vi "Teleop.vi"(10 "Match Info":T1={"Autonomous Elapsed Seconds"=0.0, "TeleOp Elapsed Seconds"=0.0, "Disabled Elapsed Seconds"=0.0, "Visited Autonomous"=FALSE, "Visited TeleOp"=FALSE, "Visited Disabled"=FALSE, "Autonomous Settings"={"Autonomous Style"=enum."Independent", "VI Refnum"=refnum}}, 11 "Call Context":T2) -> ()   [LabVIEW 2016]
doc: "This VI is called for each TeleOp packet received from the DS where the robot is not disabled. It is often used to read from the joysticks and update I/O or to update setpoints for timed control loops. It should complete and return within 20 milliseconds or it may miss DS packets."
uses:
  <vilib>/Rock Robotics/WPI/DriverStation/WPI_DriverStationDerivedRobotMode.ctl
  <vilib>/Rock Robotics/WPI/DriverStation/WPI_DriverStationMatch Info.ctl
  <vilib>/Rock Robotics/WPI/ThirdParty/CanMotor/TalonSRX/WPI_CANTalonSRX_APIControlMode.ctl
  <vilib>/Rock Robotics/WPI/Utilities/WPI_GetSetVariantRefNum.vi
  <vilib>/Rock Robotics/Network Tables/NT Write Boolean.vi
  <vilib>/Rock Robotics/Network Tables/NT Write Boolean Array.vi
  <vilib>/Rock Robotics/Network Tables/NT Write Numeric Array.vi
  <vilib>/Rock Robotics/WPI/Solenoid/Deprecated/WPI_SolenoidSetBool.vi
  <vilib>/Rock Robotics/WPI/Ultrasonic/WPI_SonarMB1010AnalogRefNum Registry Get.vi
  <vilib>/Rock Robotics/WPI/Ultrasonic/WPI_SonarMB1010AnalogGetRange.vi
  <vilib>/Rock Robotics/Network Tables/NT Read Number.vi
  <vilib>/Rock Robotics/Network Tables/NT Write Number.vi
panel:
  out "element":dbl
  out "upper limit":dbl
  out "gyro":dbl
  out "sonar distance (inches)":dbl
  out "Encoder Loop 2":string
  out "Encoder Loop":dbl
  out "Encoder Rate":dbl
  out "Encoder State":string
  out "Encoder Direction":string
  out "Distance 2":dbl
  out "Angle 2":dbl
  out "Distance":dbl
  out "Enabled":bool
  out "Compressor Running":bool
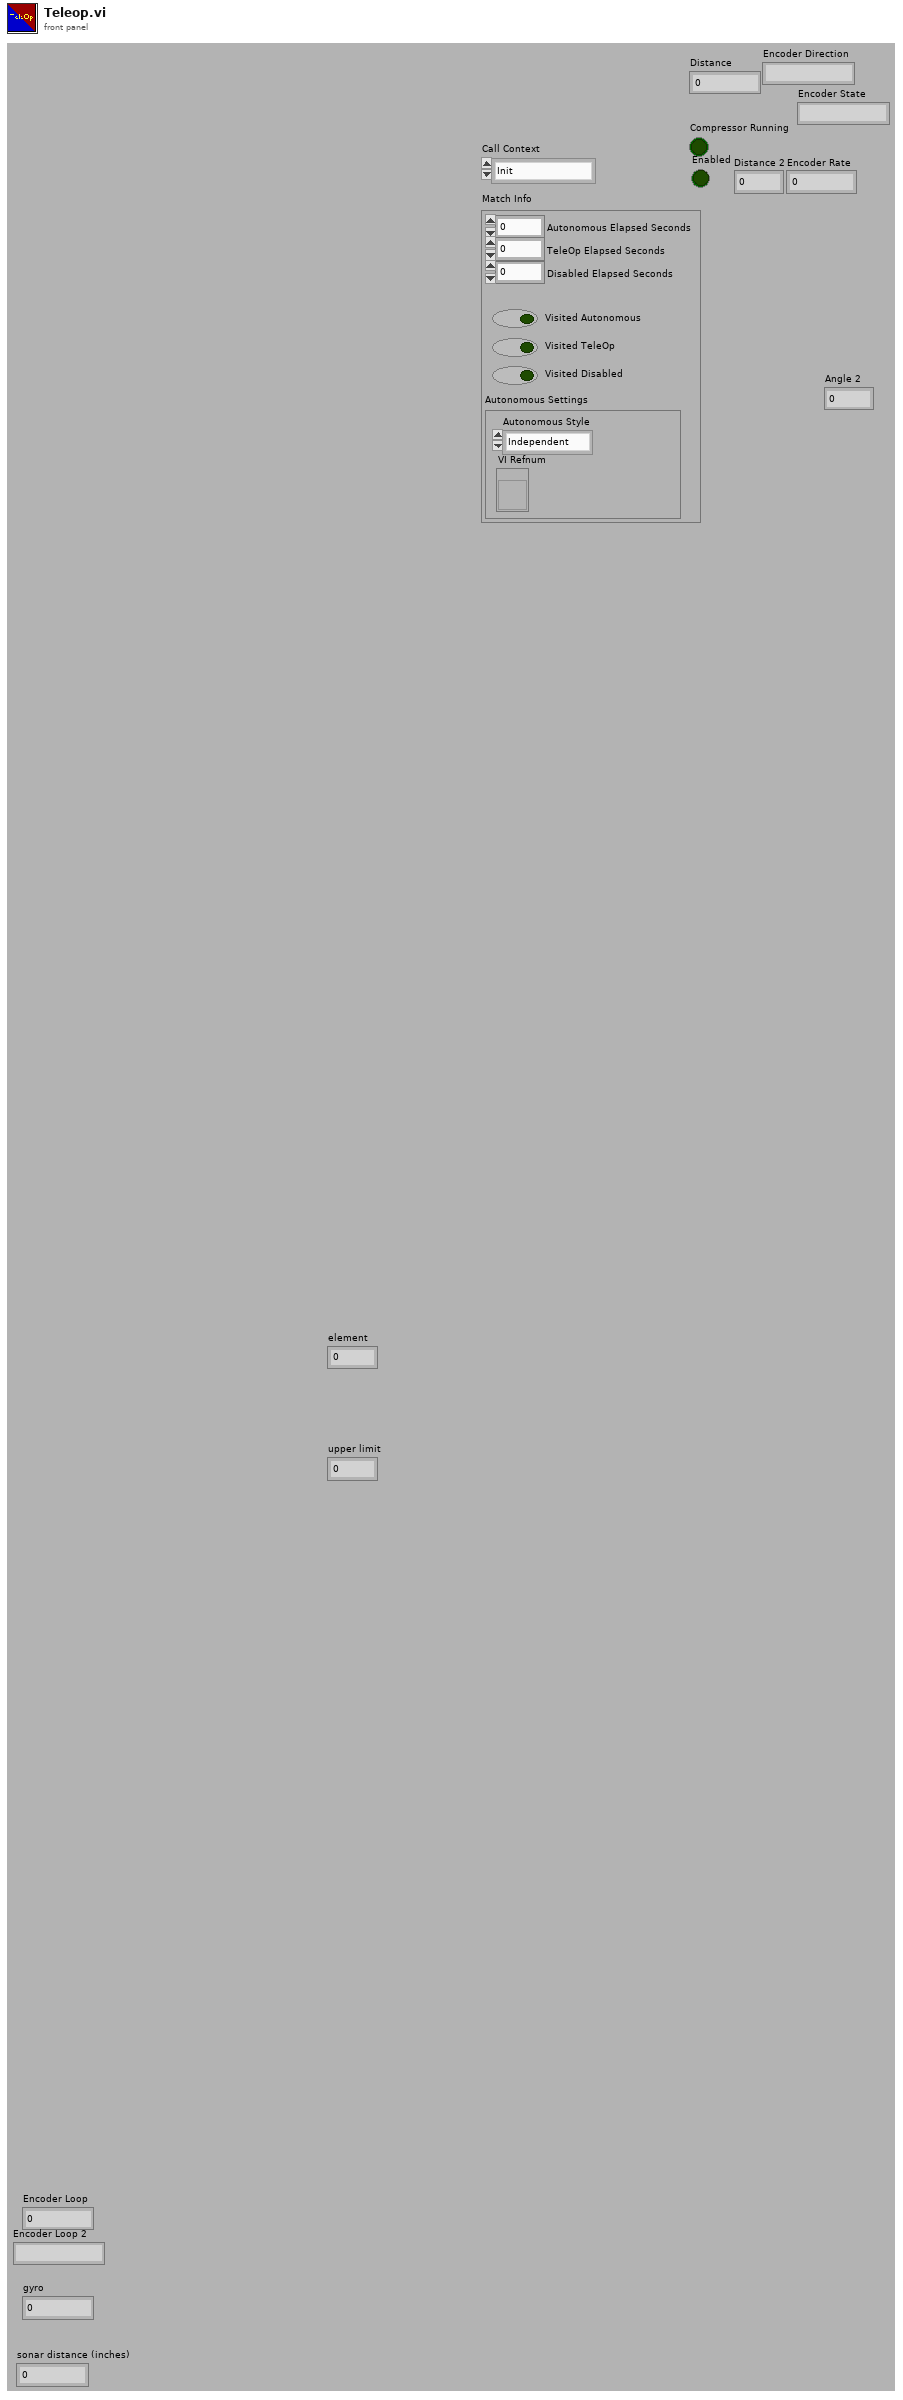
[diagram p1: front panel]
types:
  T1 = typedef "WPI_DriverStationMatch Info.ctl" = cluster{"Autonomous Elapsed Seconds":dbl, "TeleOp Elapsed Seconds":dbl, "Disabled Elapsed Seconds":dbl, "Visited Autonomous":bool, "Visited TeleOp":bool, "Visited Disabled":bool, "Autonomous Settings":cluster{"Autonomous Style":enum16{"Iterative", "Independent"}, "VI Refnum":refnum<vi>}}
  T2 = typedef "WPI_DriverStationDerivedRobotMode.ctl" = enum16{"Init", "Execute", "Stop"}
  T3 = typedef "WPI_EncoderDevRef.ctl" = cluster{"DevStatus":errorcluster, "EncoderIndex":T4, "CounterIndex":T5, "DistancePerCount":dbl, "Decoding Type":T6}
  T4 = typedef "FPGA_EncoderIdx.ctl" = enum8{"Enc 0", "Enc 1", "Enc 2", "Enc 3", "Enc 4", "Enc 5", "Enc 6", "Enc 7", "Invalid"}
  T5 = typedef "FPGA_CounterCtrSystemIndex.ctl" = enum8{"Ctr 0", "Ctr 1", "Ctr 2", "Ctr 3", "Ctr 4", "Ctr 5", "Ctr 6", "Ctr 7", "Invalid"}
  T6 = typedef "WPI_EncoderType.ctl" = enum16{"1x", "2x", "4x"}
  T7 = typedef "WPI_JoystickDevRef.ctl" = cluster{"Device":T8}
  T8 = typedef "WPI_JoystickDeviceEnum.ctl" = enum16{"USB 0", "USB 1", "USB 2", "USB 3", "USB 4", "USB 5"}
  T9 = typedef "WPI_GyroDevRef.ctl" = cluster{"DevStatus":errorcluster, "Analog Channel":T10, "Offset":dbl, "Gain (VoltsPerDegree/Second)":dbl, "Gyro Type":enum16{"Analog", "XRS450"}, "Handle":i32, "SPI Bus":T11, "Device Found":bool, "Sample Rate":dbl, "Calibrate On Open":bool}
  T10 = typedef "FPGA_AIChannel.ctl" = enum8{"AI 0", "AI 1", "AI 2", "AI 3", "AI MXP 0", "AI MXP 1", "AI MXP 2", "AI MXP 3", "Invalid"}
  T11 = typedef "spi_bus.ctl" = enum16{"SPI On-Board, CS0", "SPI On-Board, CS1", "SPI On-Board, CS2", "SPI On-Board, CS3", "SPI MXP", "Invalid"}
  T12 = typedef "WPI_SonarMB1010AnalogDeviceRef.ctl" = cluster{"AIDeviceRef":T13, "Scaling factor (V/in)":dbl, "Average Bits":u8}
  T13 = typedef "WPI_AnalogChannelDevRef.ctl" = cluster{"DevStatus":errorcluster, "Analog Channel":T10}
  T14 = typedef "WPI_CompressorDevRef.ctl" = cluster{"DevStatus":errorcluster, "Pneumatics Control Module":u8}
  T15 = typedef "WPI_SolenoidDevRef.ctl" = cluster{"DevStatus":errorcluster, "Pneumatics Control Module":u8, "Forward Solenoid Channel":T16, "Reverse Solenoid Channel":T16}
  T16 = typedef "WPI_SolenoidChannel.ctl" = enum8{"Solenoid 0", "Solenoid 1", "Solenoid 2", "Solenoid 3", "Solenoid 4", "Solenoid 5", "Solenoid 6", "Solenoid 7", "Invalid"}
  T17 = typedef "WPI_MotorControlDeviceRef.ctl" = cluster{"DeviceStatus":errorcluster, "Type":T18, "PWM":cluster{"PWM Channel":T19, "DeadBand":T20}, "CAN":cluster{"Device Number":u8, "SetOutput VI Ref":variant, "GetOutput VI Ref":variant, "Enable VI Ref":variant, "Disable VI Ref":variant, "Data":variant}, "Invert":bool}
  T18 = typedef "WPI_MotorControlType.ctl" = enum16{"PWM", "CAN"}
  T19 = typedef "FPGA_DIOPWMChannel.ctl" = enum8{"PWM 0", "PWM 1", "PWM 2", "PWM 3", "PWM 4", "PWM 5", "PWM 6", "PWM 7", "PWM 8", "PWM 9", "PWM MXP 0", "PWM MXP 1", "PWM MXP 2", "PWM MXP 3", "PWM MXP 4", "PWM MXP 5", "PWM MXP 6", "PWM MXP 7", "PWM MXP 8", "PWM MXP 9", "Invalid"}
  T20 = typedef "WPI_PWMDeadband.ctl" = cluster{"Name":string, "maxPositivePwm":i32, "minPositivePwm":i32, "centerPwm":i32, "maxNegativePwm":i32, "minNegativePwm":i32, "angularRange":u16}
  T21 = typedef "WPI_CANTalonSRX_APIControlMode.ctl" = enum8{"Percent VBus", "Speed", "Position", "Slave", "Unchanged / Invalid", "Voltage Compensation", "Current", "Motion Profile", "Motion Magic"}
  T22 = typedef "WPI_RobotDriveDevRef.ctl" = cluster{"DevStatus":errorcluster, "Motors[]":T17[], "Square Inputs":bool, "Max Output":dbl}
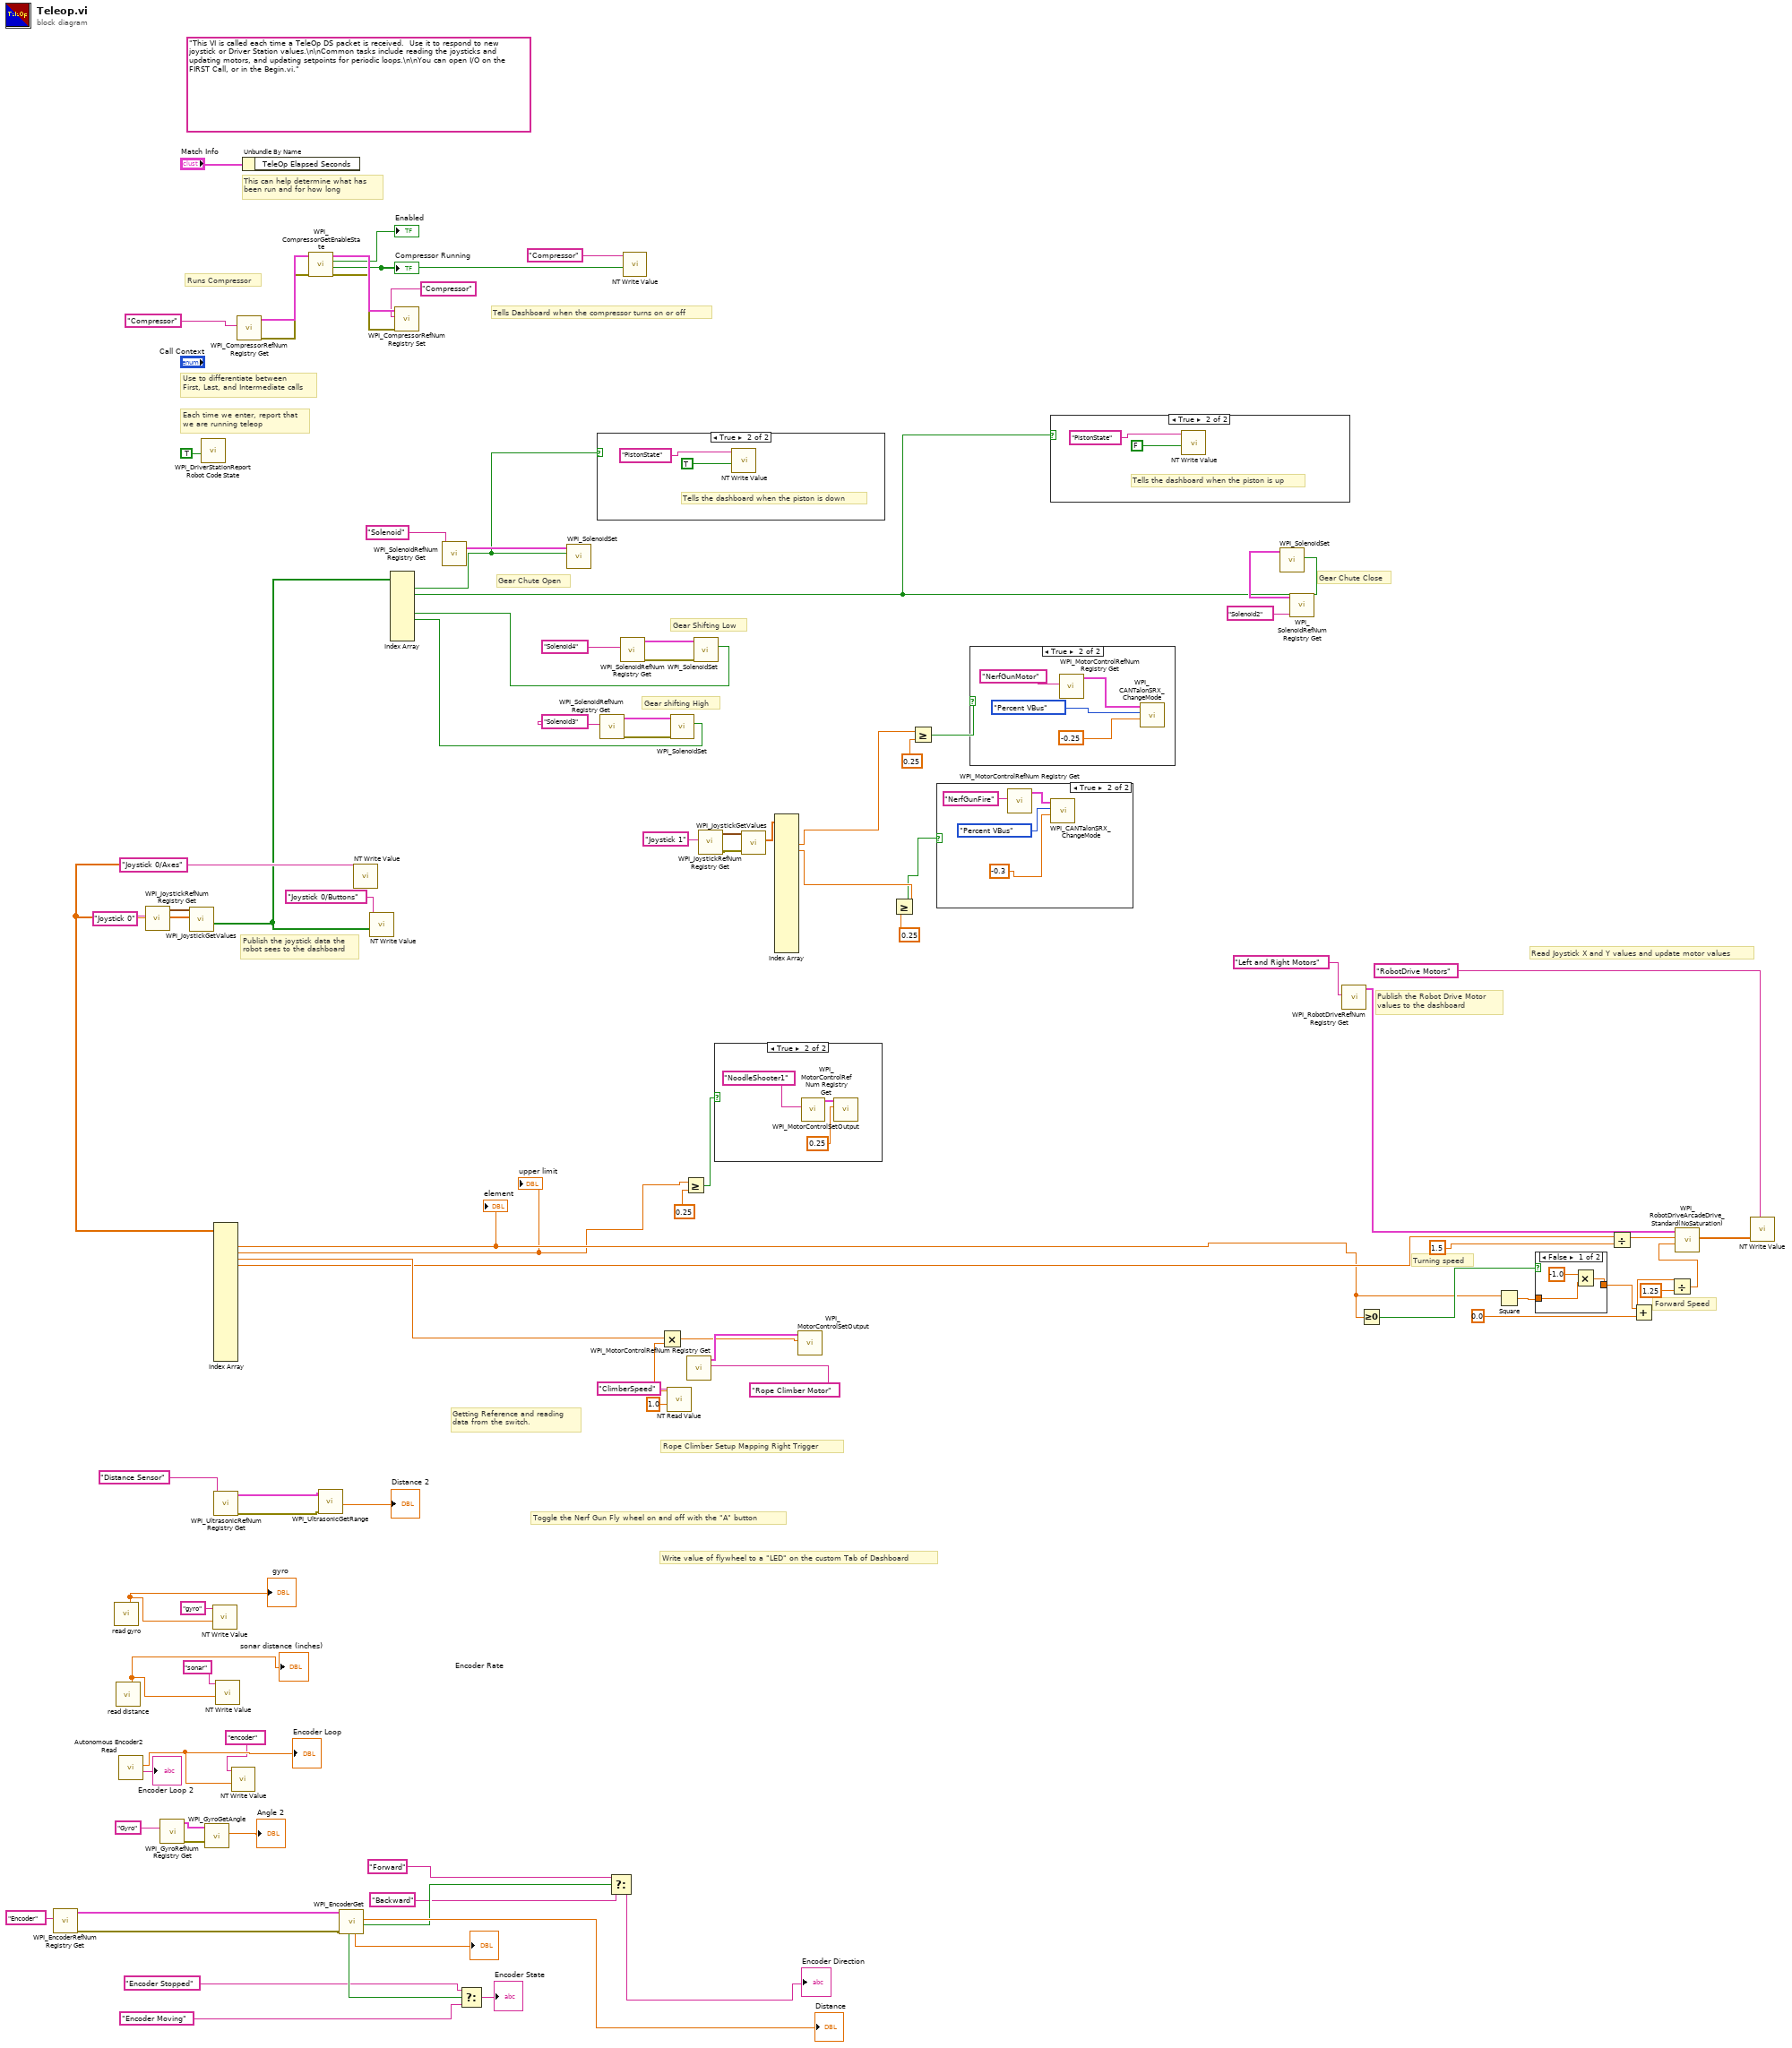
[diagram p0: block diagram]
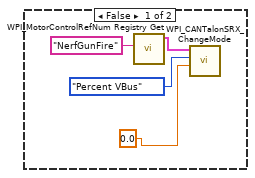
[diagram p2: hidden frame]
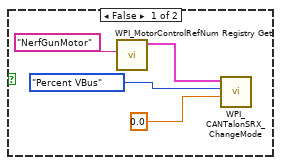
[diagram p3: hidden frame]
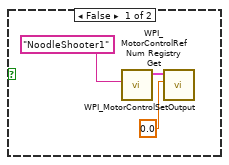
[diagram p4: hidden frame]
diagram:
  (unwired) "This VI is called each time a TeleOp DS packet is received.  Use it to respond to new joystick or Driver Station values.\n\nCommon tasks include reading the joysticks and updating motors, and updating setpoints for periodic loops.\n\nYou can open I/O on the FIRST Call, or in the Begin.vi."
  # "Write value of flywheel to a \"LED\" on the custom Tab of Dashboard"
  # "Toggle the Nerf Gun Fly wheel on and off with the \"A\" button"
  # "Gear Chute Open"
  # "Gear Chute Close"
  # "Gear shifting High"
  # "Gear Shifting Low"
  # "Turning speed"
  # "Forward Speed"
  # "Rope Climber Setup Mapping Right Trigger"
  # "Getting Reference and reading \ndata from the switch."
  # "Publish the joystick data the\nrobot sees to the dashboard"
  # "Publish the Robot Drive Motor\nvalues to the dashboard"
  # "Read Joystick X and Y values and update motor values"
  # "Tells Dashboard when the compressor turns on or off"
  # "Runs Compressor"
  # "Each time we enter, report that\nwe are running teleop"
  # "Use to differentiate between\nFirst, Last, and Intermediate calls"
  # "This can help determine what has\nbeen run and for how long"
  n1 = call <vilib>:"WPI_EncoderRefNum Registry Get.vi"("refnum name"="Encoder") -> ("error out"=w63:errorcluster, "EncoderDevRef"=w64:T3)  [unwired: 9 in]
  n2 = call "read gyro.vi"() -> ("Angle 2"=w36:dbl)  [unwired: 10 in, 1 out]
  "gyro" <- w36
  n3 = call "read distance.vi"() -> ("Distance 2"=w34:dbl)  [unwired: 10 in, 1 out]
  "sonar distance (inches)" <- w34
  n4 = call "Autonomous Encoder2 Read.vi"() -> ("Encoder Direction"=→"Encoder Loop 2":string, "Encoder Distance"=w31:dbl)  [unwired: 9 in, 1 out]
  "Encoder Loop" <- w31
  n5 = call <vilib>:"WPI_JoystickRefNum Registry Get.vi"("refnum name"="Joystick 0") -> ("JoystickDevRef"=w80:T7)  [unwired: 1 in, 9 out]
  n6 = call <vilib>:"WPI_GyroRefNum Registry Get.vi"("refnum name"="Gyro") -> ("error out"=w58:errorcluster, "GyroDevRef"=w59:T9)  [unwired: 9 in]
  n7 = call <vilib>:"WPI_JoystickGetValues.vi"("JoystickDevRef"=w80) -> ("Buttons"=w74:bool[], "Axes"=w77:dbl[])  [unwired: 6 in, 3 out]
  n8 = call <vilib>:"WPI_DriverStationReport Robot Code State.vi"("TeleOp"=TRUE ("Autonomous")) -> ()  [unwired: 10 in, 1 out]
  n9 = call <vilib>:"WPI_GyroGetAngle.vi"("error in"=w58, "GyroDevRef"=w59) -> ("Angle"=→"Angle 2":dbl)  [unwired: 5 in, 4 out]
  n10 = call-poly <vilib>:"NT Write Value.vi"("Numeric"=w36, "Name"="gyro") -> ()  [unwired: 9 in, 1 out]
  n11 = Index Array(array=w77) -> (element #2=w29:dbl, element #3=w9:dbl, element #4=w68:dbl, element #5=w44:dbl)  [unwired: 20 in, 16 out]
  "upper limit" <- w9
  "element" <- w29
  n12 = call-poly <vilib>:"WPI_UltrasonicRefNum Registry Get.vi"("refnum name"="Distance Sensor") -> ("error out"=w54:errorcluster, "SonarMB1010AnalogDevRef"=w56:T12)  [unwired: 9 in]
  n13 = call-poly <vilib>:"NT Write Value.vi"("Numeric"=w34, "Name"="sonar") -> ()  [unwired: 9 in, 1 out]
  n14 = call-poly <vilib>:"NT Write Value.vi"("Numeric"=w31, "Name"="encoder") -> ()  [unwired: 9 in, 1 out]
  n15 = call <vilib>:"WPI_CompressorRefNum Registry Get.vi"("refnum name"="Compressor") -> ("error out"=w90:errorcluster, "CompressorDevRef"=w92:T14)  [unwired: 9 in]
  n16 = Unbundle By Name("Match Info") -> ()  [unwired: 1 out]
  n17 = call <vilib>:"WPI_CompressorGetEnableState.vi"("error in (no error)"=w90, "CompressorDevRef"=w92) -> ("error out"=w89:errorcluster, "Compressor Running"=w84:bool, "Enabled"=→"Enabled":bool, "CompressorDevRef"=w91:T14)  [unwired: 6 in]
  "Compressor Running" <- w84
  n18 = call-poly <vilib>:"WPI_UltrasonicGetRange.vi"("error in"=w54, "SonarMB1010AnalogDevRef"=w56) -> ("Distance"=→"Distance 2":dbl)  [unwired: 7 in, 2 out]
  n19 = call <vilib>:"WPI_EncoderGet.vi"("error in (no error)"=w63, "EncoderDevRef"=w64) -> ("Direction"=w53:bool, "Distance"=→"Distance":dbl, "Rate"=→"Encoder Rate":dbl, "Stopped"=w49:bool)  [unwired: 4 in, 2 out]
  n20 = call-poly <vilib>:"NT Write Value.vi"("Numeric Array"=w77, "Name"="Joystick 0/Axes") -> ()  [unwired: 9 in, 1 out]
  n21 = call-poly <vilib>:"NT Write Value.vi"("Boolean Array"=w74, "Name"="Joystick 0/Buttons") -> ()  [unwired: 9 in, 1 out]
  n22 = Index Array(array=w74) -> (element #1=w69:bool, element #2=w10:bool, element #5=w21:bool, element #6=w22:bool)  [unwired: 9 in, 5 out]
  n23 = call <vilib>:"WPI_CompressorRefNum Registry Set.vi"("error in (no error)"=w89, "refnum name"="Compressor", "CompressorDevRef"=w91) -> ()  [unwired: 7 in, 2 out]
  n24 = call <vilib>:"WPI_SolenoidRefNum Registry Get.vi"("refnum name"="Solenoid") -> ("SolenoidDevRef"=w70:T15)  [unwired: 9 in, 1 out]
  n25 = Select(t="Encoder Stopped", s=w49, f="Encoder Moving") -> (s? t:f=→"Encoder State":string)
  n26 = call-poly <vilib>:"WPI_SolenoidSet.vi"("Value"=w69, "SolenoidDevRef"=w70) -> ()  [unwired: 8 in, 2 out]
  n27 = case shown="True" w69 {
    frame False {
    }
    frame True {
      # "Tells the dashboard when the piston is down"
      n28 = call-poly <vilib>:"NT Write Value.vi"("Boolean"=TRUE, "Name"="PistonState") -> ()  [unwired: 9 in, 1 out]
    }
  }
  n29 = call <vilib>:"WPI_SolenoidRefNum Registry Get.vi"("refnum name"="Solenoid3") -> ("error out"=w15:errorcluster, "SolenoidDevRef"=w17:T15)  [unwired: 9 in]
  n30 = Select(t="Forward", s=w53, f="Backward") -> (s? t:f=→"Encoder Direction":string)
  n31 = call <vilib>:"WPI_SolenoidRefNum Registry Get.vi"("refnum name"="Solenoid4") -> ("error out"=w18:errorcluster, "SolenoidDevRef"=w20:T15)  [unwired: 9 in]
  n32 = call-poly <vilib>:"NT Write Value.vi"("Boolean"=w84, "Name"="Compressor") -> ()  [unwired: 9 in, 1 out]
  n33 = call-poly <vilib>:"NT Read Value.vi"("Default Value"=1.0, "Name"="ClimberSpeed") -> ("Numeric"=w25:dbl)  [unwired: 8 in, 1 out]
  n34 = Multiply(x=w68, y=w25) -> (x*y=w24:dbl)
  n35 = call-poly <vilib>:"WPI_SolenoidSet.vi"("error in (no error)"=w15, "Value"=w22, "SolenoidDevRef"=w17) -> ()  [unwired: 7 in, 2 out]
  n36 = Greater Or Equal?(x=w9, y=0.25 ("x")) -> (x >= y?=w8:bool)
  n37 = call <vilib>:"WPI_MotorControlRefNum Registry Get.vi"("refnum name"="Rope Climber Motor") -> ("MotorControlDevRef"=w27:T17)  [unwired: 9 in, 1 out]
  n38 = call-poly <vilib>:"WPI_SolenoidSet.vi"("error in (no error)"=w18, "Value"=w21, "SolenoidDevRef"=w20) -> ()  [unwired: 7 in, 2 out]
  n39 = call <vilib>:"WPI_JoystickRefNum Registry Get.vi"("refnum name"="Joystick 1") -> ("error out"=w11:errorcluster, "JoystickDevRef"=w13:T7)  [unwired: 1 in, 8 out]
  n40 = case shown="True" w8 {
    frame False {
      n41 = call <vilib>:"WPI_MotorControlRefNum Registry Get.vi"("refnum name"="NoodleShooter1") -> ("MotorControlDevRef"=w98:T17)  [unwired: 9 in, 1 out]
      n42 = call <vilib>:"WPI_MotorControlSetOutput.vi"("Output"=0.0, "MotorControlDevRef"=w98) -> ()  [unwired: 7 in, 3 out]
    }
    frame True {
      n43 = call <vilib>:"WPI_MotorControlRefNum Registry Get.vi"("refnum name"="NoodleShooter1") -> ("MotorControlDevRef"=w101:T17)  [unwired: 9 in, 1 out]
      n44 = call <vilib>:"WPI_MotorControlSetOutput.vi"("Output"=0.25, "MotorControlDevRef"=w101) -> ()  [unwired: 7 in, 3 out]
    }
  }
  n45 = call <vilib>:"WPI_JoystickGetValues.vi"("error in (no error)"=w11, "JoystickDevRef"=w13) -> ("Axes"=w12:dbl[])  [unwired: 5 in, 4 out]
  n46 = Index Array(array=w12) -> (element #3=w5:dbl, element #4=w3:dbl)  [unwired: 20 in, 18 out]
  n47 = call <vilib>:"WPI_MotorControlSetOutput.vi"("Output"=w24, "MotorControlDevRef"=w27) -> ()  [unwired: 7 in, 3 out]
  n48 = Greater Or Equal?(x=w3, y=0.25 ("x")) -> (x >= y?=w1:bool)
  n49 = Greater Or Equal?(x=w5, y=0.25 ("x")) -> (x >= y?=w4:bool)
  n50 = case shown="True" w1 {
    frame False {
      n51 = call <vilib>:"WPI_MotorControlRefNum Registry Get.vi"("refnum name"="NerfGunFire") -> ("MotorControlDevRef"=w103:T17)  [unwired: 9 in, 1 out]
      n52 = call <vilib>:"WPI_CANTalonSRX_ChangeMode.vi"("Output"=0.0, "Control Mode"=WPI_CANTalonSRX_APIControlMode."Percent VBus", "CAN Talon SRX Ref"=w103) -> ()  [unwired: 7 in, 2 out]
    }
    frame True {
      n53 = call <vilib>:"WPI_MotorControlRefNum Registry Get.vi"("refnum name"="NerfGunFire") -> ("MotorControlDevRef"=w109:T17)  [unwired: 9 in, 1 out]
      n54 = call <vilib>:"WPI_CANTalonSRX_ChangeMode.vi"("Output"=-0.3, "Control Mode"=WPI_CANTalonSRX_APIControlMode."Percent VBus", "CAN Talon SRX Ref"=w109) -> ()  [unwired: 7 in, 2 out]
    }
  }
  n55 = case shown="True" w4 {
    frame False {
      n56 = call <vilib>:"WPI_MotorControlRefNum Registry Get.vi"("refnum name"="NerfGunMotor") -> ("MotorControlDevRef"=w114:T17)  [unwired: 9 in, 1 out]
      n57 = call <vilib>:"WPI_CANTalonSRX_ChangeMode.vi"("Output"=0.0, "Control Mode"=WPI_CANTalonSRX_APIControlMode."Percent VBus", "CAN Talon SRX Ref"=w114) -> ()  [unwired: 7 in, 2 out]
    }
    frame True {
      n58 = call <vilib>:"WPI_MotorControlRefNum Registry Get.vi"("refnum name"="NerfGunMotor") -> ("MotorControlDevRef"=w118:T17)  [unwired: 9 in, 1 out]
      n59 = call <vilib>:"WPI_CANTalonSRX_ChangeMode.vi"("Output"=-0.25, "Control Mode"=WPI_CANTalonSRX_APIControlMode."Percent VBus", "CAN Talon SRX Ref"=w118) -> ()  [unwired: 7 in, 2 out]
    }
  }
  n60 = case shown="True" w10 {
    frame False {
    }
    frame True {
      # "Tells the dashboard when the piston is up"
      n61 = call-poly <vilib>:"NT Write Value.vi"("Boolean"=FALSE, "Name"="PistonState") -> ()  [unwired: 9 in, 1 out]
    }
  }
  n62 = call <vilib>:"WPI_SolenoidRefNum Registry Get.vi"("refnum name"="Solenoid2") -> ("SolenoidDevRef"=w72:T15)  [unwired: 9 in, 1 out]
  n63 = call-poly <vilib>:"WPI_SolenoidSet.vi"("Value"=w10, "SolenoidDevRef"=w72) -> ()  [unwired: 8 in, 2 out]
  n64 = call <vilib>:"WPI_RobotDriveRefNum Registry Get.vi"("refnum name"="Left and Right Motors") -> ("RobotDriveDevRef"=w82:T22)  [unwired: 1 in, 9 out]
  n65 = Greater Or Equal To 0?(x=w29) -> (x >= 0?=w39:bool)
  n66 = Square(x=w29) -> (x^2=w38:dbl)
  n67 = case shown="False" w39 {
    tunnel: w38 -> [w123 w124]
    tunnel: [w121 w124] -> w37
    frame False {
      n68 = Multiply(x=-1.0, y=w123) -> (x*y=w121:dbl)
    }
    frame True {
    }
  }
  n69 = Divide(x=w44, y=1.5) -> (x/y=w66:dbl)
  n70 = Add(x=w37, y=0.0) -> (x+y=w41:dbl)
  n71 = Divide(x=w41, y=1.25) -> (x/y=w40:dbl)
  n72 = call <vilib>:"WPI_RobotDriveArcadeDrive_Standard(NoSaturation).vi"("Y axis value"=w40, "X axis value"=w66, "RobotDriveDevRef"=w82) -> ("Motor Values"=w76:dbl[])  [unwired: 1 in, 7 out]
  n73 = call-poly <vilib>:"NT Write Value.vi"("Numeric Array"=w76, "Name"="RobotDrive Motors") -> ()  [unwired: 9 in, 1 out]
